vi "Evn-settings.vi"(7 "setting type":T1) -> ()   [LabVIEW 2019]
uses:
  hwsetting.ctl
  _ctrl/rw.ctl
  _ctrl/BP4610_config.ctl
  _ctrl/DSP_config.ctl
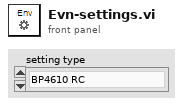
[diagram p1: front panel]
types:
  T1 = typedef "hwsetting.ctl" = enum16{"BP4610 RC", "DSP1500 RC", "AO"}
  T2 = typedef "BP4610_config.ctl" = cluster{"VISA":refnum<visa-resource-name>, "Limit-BP":cluster{"Set":enum16{"Current", "Voltage"}, "Voltage+[V]":dbl, "Current+[A]":dbl, "Voltage-[V]":dbl, "Current-[A]":dbl}, "SET BP":cluster{"Set":enum16{"Current", "Voltage", "FREQ/WAVE"}, "Operation mode":u16, "Voltage[Vp-p]":dbl, "Current[Ap-p]":dbl, "Voltage[V]":dbl, "Current[A]":dbl, "Frequency[Hz]":dbl, "Waveform":enum16{"Sine", "Square", "ARB 1", "ARB 2", "ARB 3", "ARB 4", "ARB 5", "ARB 6", "ARB 7", "ARB 8", "ARB 9", "ARB 10", "ARB 11", "ARB 12", "ARB 13", "ARB 14", "ARB 15", "ARB 16"}}}
  T3 = typedef "rw.ctl" = enum16{"read", "write"}
  T4 = typedef "DSP_config.ctl" = cluster{"Port":refnum<visa-resource-name>, "OVP Level":dbl, "OCP Level":dbl, "Current":dbl, "Voltage":dbl}
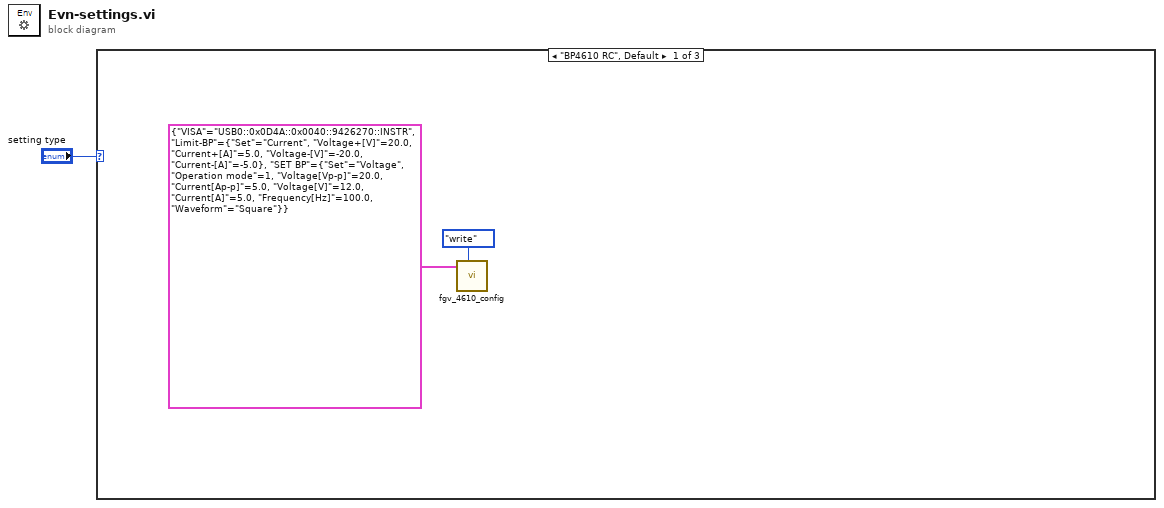
[diagram p0: block diagram]
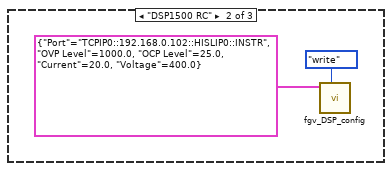
[diagram p2: hidden frame]
diagram:
  n1 = case shown="\"BP4610 RC\", Default" "setting type" {
    frame "BP4610 RC", Default {
      n2 = call "fgv_4610_config.vi"("cmd"=rw."write", "BP4610 Config"=T2 {"VISA"="USB0::0x0D4A::0x0040::9426270::INSTR", "Limit-BP"={"Set"=enum."Current", "Voltage+[V]"=20.0, "Current+[A]"=5.0, "Voltage-[V]"=-20.0, "Current-[A]"=-5.0}, "SET BP"={"Set"=enum."Voltage", "Operation mode"=1, "Voltage[Vp-p]"=20.0, "Current[Ap-p]"=5.0, "Voltage[V]"=12.0, "Current[A]"=5.0, "Frequency[Hz]"=100.0, "Waveform"=enum."Square"}} ("BP4610 Config 2")) -> ()  [unwired: 8 in, 2 out]
    }
    frame "DSP1500 RC" {
      n3 = call "fgv_DSP_config.vi"("cmd"=rw."write", "DSP Config HV IN"=T4 {"Port"="TCPIP0::192.168.0.102::HISLIP0::INSTR", "OVP Level"=1000.0, "OCP Level"=25.0, "Current"=20.0, "Voltage"=400.0} ("DSP1950 Config 2")) -> ()  [unwired: 7 in, 3 out]
    }
    frame "AO" {
    }
  }
